vi "Get Address.vi"(4 "Instrument Info":T1) -> (1 "Address":string)   [LabVIEW 2018]
uses:
  Station/Station Support/Controls/Instrument Info.ctl
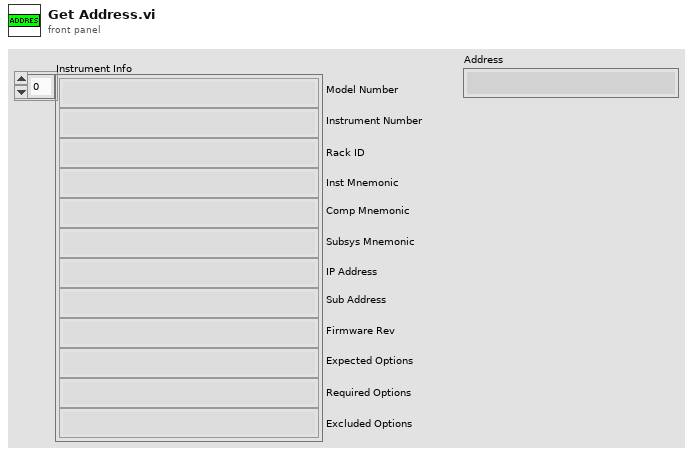
[diagram p1: front panel]
types:
  T1 = typedef "Instrument Info.ctl" = string[]
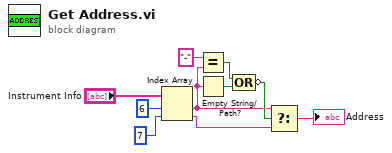
[diagram p0: block diagram]
diagram:
  n1 = Index Array(array="Instrument Info", index #1=6 ("index"), index #2=7 ("index")) -> (element #1=w3:string, element #2=w1:string)
  n2 = Equal?(x="-", y=w3) -> (x = y?=w5:bool)
  n3 = Empty String/Path?(string/path=w3) -> (empty?=w4:bool)
  n4 = Compound Arithmetic op=OR(w5, w4) -> (invert w6:bool)
  n5 = Select(t=w3, s=w6, f=w1) -> (s? t:f=→"Address":string)
